vi "main - demo lvORM.vi"() -> ()   [LabVIEW 2018]
uses:
  _Serializable Base Object/_ISerializable.lvclass
  demo/Implementations/Component-A.lvclass
  U:/repos/modules/lv-orm/_Serializable Base Object/_ISerializable.lvclass
  demo/Implementations/Component-B.lvclass
  demo/Implementations/Product-A.lvclass
  demo/Implementations/Product-B.lvclass
  ORM/LV-ORM.lvclass
panel:
  out "all obj":refnum<class "_ISerializable.lvclass">[](array[class])
  in  "class":string(combo)
  in  "listbox":i32(listbox) caption="<< CLASSNAME >>"
  in  "add":bool
  in  "edit":bool
  in  "del":bool
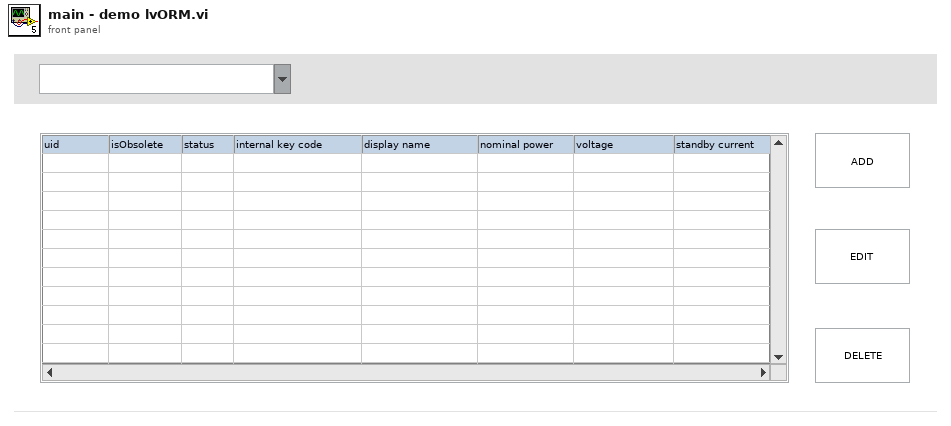
[diagram p1: front panel]
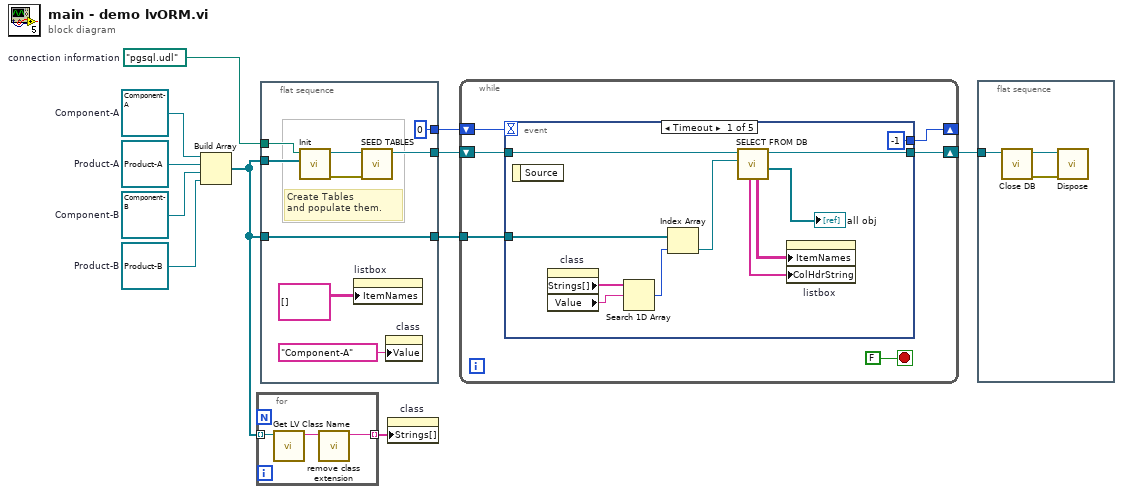
[diagram p0: block diagram]
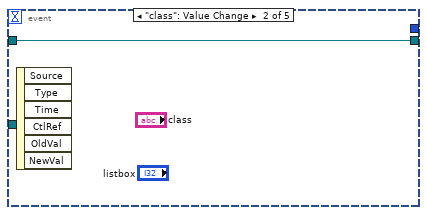
[diagram p2: hidden frame]
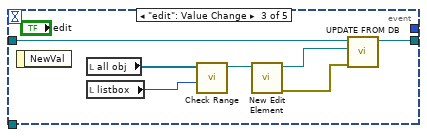
[diagram p3: hidden frame]
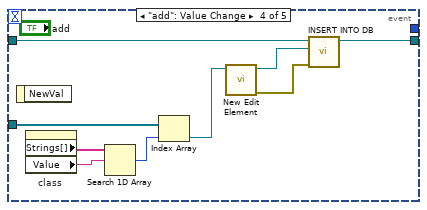
[diagram p4: hidden frame]
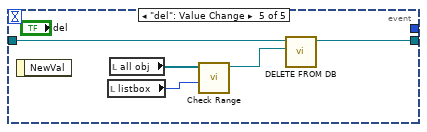
[diagram p5: hidden frame]
diagram:
  w1 = path "pgsql.udl"  # connection information
  w5 = refnum<class "Product-B.lvclass"> refnum  # Product-B
  w8 = refnum<class "Product-A.lvclass"> refnum  # Product-A
  w6 = refnum<class "Component-B.lvclass"> refnum  # Component-B
  w7 = refnum<class "Component-A.lvclass"> refnum  # Component-A
  n1 = Build Array(w7, w8, w6, w5) -> (w4:refnum<class "_ISerializable.lvclass">[])
  n2 = for {
    tunnel: w4 -> [w13] mode=indexing
    tunnel: [w12] -> w3 mode=indexing
    n3 = call <vilib>:"Get LV Class Name.vi"("object"=w13) -> ("class name"=w14:string)  [unwired: 9 in, 1 out]
    n4 = call "remove class extension.vi"("class name in"=w14) -> ("class name out"=w12:string)  [unwired: 10 in]
  }
  n5 = flat-sequence {
    tunnel: [w16] -> w11
    tunnel: w4 -> [w20]
    tunnel: w4 -> [w19]
    tunnel: [w19] -> w9
    tunnel: [0] -> w2
    tunnel: w1 -> [w15]
    frame #0 {
      # "Create Tables\nand populate them."
      n6 = call "Init.vi"("Array"=w20, "connection information"=w15) -> ("error out"=w21:errorcluster, "LV-ORM out"=w22:refnum<class "LV-ORM.lvclass">)  [unwired: 8 in]
      n7 = property on="listbox" class="MCListbox (strict)"("ItemNames"=string[][] []) -> ()  [unwired: 2 in, 2 out]
      n8 = call "SEED TABLES.vi"("error in"=w21, "LV-ORM in"=w22) -> ("LV-ORM out"=w16:refnum<class "LV-ORM.lvclass">)  [unwired: 8 in, 1 out]
      n9 = property on="class" class="CmbBox"("Value"="Component-A" ("Component-A")) -> ()  [unwired: 2 in, 2 out]
    }
  }
  n10 = property on="class" class="CmbBox"("Strings[]"=w3) -> ()  [unwired: 2 in, 2 out]
  n11 = while {
    shift-right: [w28] -> w10
    shift-left: w11 -> [w29]
    tunnel: w9 -> [w26]
    shift-right: [w24] -> _
    shift-left: w2 -> [w25]
    stop <- FALSE stop-if-true
    n12 = event shown="[0] Timeout" {
      selector: _ -> [_ _ _ _ _]
      dyn-events: _ -> [_ _ _ _ _]
      timeout: w25 -> [_ _ _ _ _]
      tunnel: w29 -> [w40 w41 w42 w57 w62]
      tunnel: [w39 w41 w48 w56 w61] -> w28
      tunnel: w26 -> [w36 _ _ w50 _]
      tunnel: [-1 _ _ _ _] -> w24
      event Timeout {
        n13 = event-data() -> ()  [unwired: 1 in, 1 out]
        n14 = property on="class" class="CmbBox"() -> ("Strings[]"=w38:string[], "Value"=w31:string)  [unwired: 2 in, 2 out]
        n15 = Search 1D Array(1D array=w38, element=w31) -> (index of element=w37:i32)  [unwired: 1 in]
        n16 = Index Array(array=w36, index=w37) -> (element=w35:refnum<class "_ISerializable.lvclass">)
        n17 = call "SELECT FROM DB.vi"("object"=w35, "orm in"=w40) -> ("all obj"=→"all obj":refnum<class "_ISerializable.lvclass">[], "orm out"=w39:refnum<class "LV-ORM.lvclass">, "data"=w34:string[][], "column names"=w30:string[])  [unwired: 5 in, 1 out]
        n18 = property on="listbox" class="MCListbox (strict)"("ItemNames"=w34, "ColHdrString"=w30) -> ()  [unwired: 2 in, 2 out]
      }
      event "class": Value Change {
        n19 = event-data() -> ()  [unwired: 1 in, 6 out]
      }
      event "edit": Value Change {
        n20 = event-data() -> ()  [unwired: 1 in, 1 out]
        n21 = local read "all obj"() -> (w44:refnum<class "_ISerializable.lvclass">[])
        n22 = local read "listbox"() -> (w43:i32)
        n23 = call "Check Range.vi"("listbox"=w43, "all obj"=w44) -> ("_ISerializable out"=w45:refnum<class "_ISerializable.lvclass">)  [unwired: 9 in]
        n24 = call-dynamic "New Edit Element.vi"("_ISerializable in"=w45) -> ("error out"=w46:errorcluster, "_ISerializable out"=w47:refnum<class "_ISerializable.lvclass">)  [unwired: 9 in]
        n25 = call "UPDATE FROM DB.vi"("error in"=w46, "object"=w47, "orm in"=w42) -> ("orm out"=w48:refnum<class "LV-ORM.lvclass">)  [unwired: 7 in, 1 out]
      }
      event "add": Value Change {
        n26 = event-data() -> ()  [unwired: 1 in, 1 out]
        n27 = property on="class" class="CmbBox"() -> ("Strings[]"=w52:string[], "Value"=w53:string)  [unwired: 2 in, 2 out]
        n28 = Search 1D Array(1D array=w52, element=w53) -> (index of element=w51:i32)  [unwired: 1 in]
        n29 = Index Array(array=w50, index=w51) -> (element=w49:refnum<class "_ISerializable.lvclass">)
        n30 = call-dynamic "New Edit Element.vi"("_ISerializable in"=w49) -> ("error out"=w54:errorcluster, "_ISerializable out"=w55:refnum<class "_ISerializable.lvclass">)  [unwired: 9 in]
        n31 = call "INSERT INTO DB.vi"("error in"=w54, "object"=w55, "orm in"=w57) -> ("orm out"=w56:refnum<class "LV-ORM.lvclass">)  [unwired: 7 in, 1 out]
      }
      event "del": Value Change {
        n32 = event-data() -> ()  [unwired: 1 in, 1 out]
        n33 = local read "listbox"() -> (w59:i32)
        n34 = local read "all obj"() -> (w60:refnum<class "_ISerializable.lvclass">[])
        n35 = call "Check Range.vi"("listbox"=w59, "all obj"=w60) -> ("_ISerializable out"=w58:refnum<class "_ISerializable.lvclass">)  [unwired: 9 in]
        n36 = call "DELETE FROM DB.vi"("object"=w58, "orm in"=w62) -> ("orm out"=w61:refnum<class "LV-ORM.lvclass">)  [unwired: 8 in, 1 out]
      }
    }
  }
  n37 = flat-sequence {
    tunnel: w10 -> [w65]
    frame #0 {
      n38 = call "Close DB.vi"("LV-ORM in"=w65) -> ("error out"=w63:errorcluster, "LV-ORM out"=w64:refnum<class "LV-ORM.lvclass">)  [unwired: 9 in]
      n39 = call "Dispose.vi"("error in (no error)"=w63, "LV-ORM in"=w64) -> ()  [unwired: 9 in, 1 out]
    }
  }
